vi "Mean and STD.vi"(0 "Data (in)":dbl[][](array[numeric]) format="%.2f", 11 "Number of Impulses":i32) -> (4 "Mean and STD":dbl[][](graph), 10 "Mean":dbl[][](array[numeric]) format="%.2f", 15 "STD":dbl[][](array[numeric]) format="%.2f")   [LabVIEW 2016, in "stats.lvlib"]
uses:
  stats.lvlib
  nan operations/nan operations.lvlib
panel:
  # "Copyright Americo A. Migliaccio (c) 2002 All Rights Reserved by Author"
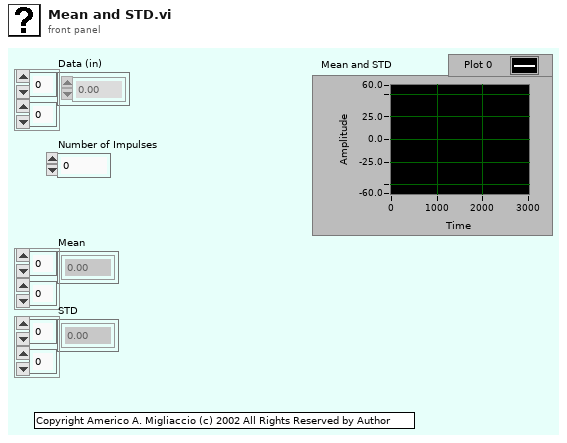
[diagram p1: front panel]
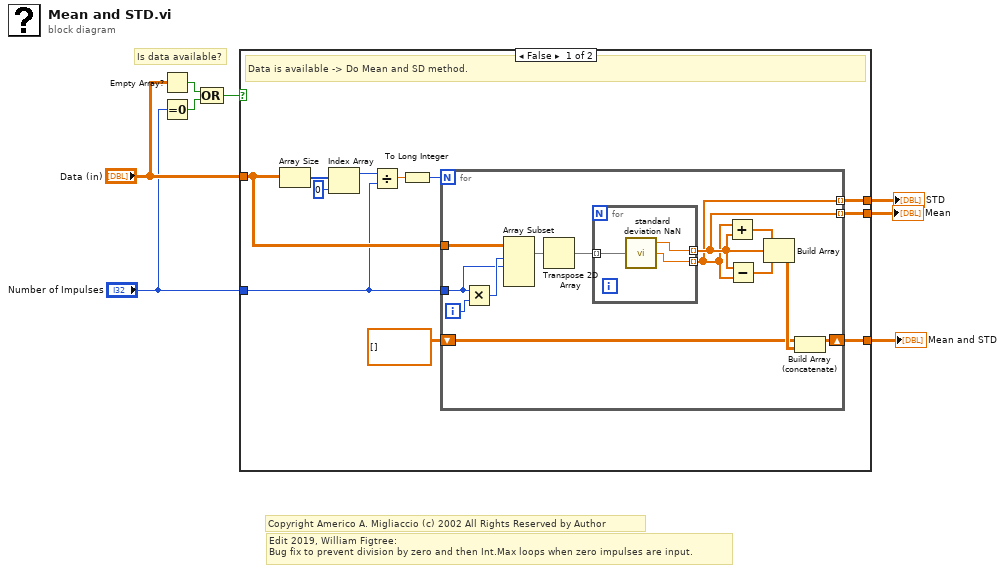
[diagram p0: block diagram]
diagram:
  # "Is data available?"
  # "Edit 2019, William Figtree:\nBug fix to prevent division by zero and then Int.Max loops when zero impulses are input."
  # "Copyright Americo A. Migliaccio (c) 2002 All Rights Reserved by Author"
  n1 = Empty Array?(array="Data (in)") -> (empty?=w3:bool)
  n2 = Equal To 0?(x="Number of Impulses") -> (x = 0?=w2:bool)
  n3 = Compound Arithmetic op=OR(w3, w2) -> (w1:bool)
  n4 = case shown="False" w1 {
    tunnel: "Data (in)" -> [w14 _]
    tunnel: "Number of Impulses" -> [w13 _]
    tunnel: [w11 _] -> w8
    tunnel: [w10 _] -> w7
    tunnel: [w9 _] -> w6
    frame False {
      # "Data is available -> Do Mean and SD method."
      n5 = Array Size(array=w14) -> (size(s)=w19:i32[])
      n6 = Index Array(array=w19, index=0 ("Index")) -> (element=w17:i32)
      n7 = Divide(x=w17, y=w13) -> (x/y=w16:dbl)
      n8 = To Long Integer(number=w16) -> (32bit integer=w15:i32)
      n9 = for {
        N: w15 -> [_]
        tunnel: w14 -> [w32]
        tunnel: w13 -> [w28]
        shift-right: [w23] -> w11
        shift-left: dbl[][] [] -> [w22]
        tunnel: [w21] -> w10 mode=indexing
        tunnel: [w20] -> w9 mode=indexing
        i -> [w30]
        n10 = Multiply(x=w28, y=w30) -> (x*y=w29:i32)
        n11 = Array Subset(array=w32, index (row)=w29, length (row)=w28) -> (w31:dbl[][])  [unwired: 2 in]
        n12 = Transpose 2D Array(2D array=w31) -> (transposed array=w27:dbl[][])
        n13 = for {
          tunnel: w27 -> [w35] mode=indexing
          tunnel: [w34] -> w21 mode=indexing
          tunnel: [w33] -> w20 mode=indexing
          n14 = call "standard deviation NaN.vi"("Array"=w35) -> ("standard deviation"=w33:dbl, "mean"=w34:dbl)  [unwired: 2 in, 1 out]
        }
        n15 = Add(x=w20, y=w21) -> (x+y=w26:dbl[])
        n16 = Subtract(x=w21, y=w20) -> (x-y=w25:dbl[])
        n17 = Build Array(w26, w21, w25) -> (w24:dbl[][])
        n18 = Build Array (concatenate)(w22, w24) -> (w23:dbl[][])
      }
    }
    frame True {
      # "Data is not available. Return nothing."
    }
  }
  "Mean and STD" <- w8
  "Mean" <- w7
  "STD" <- w6
